vi "12_2.vi"() -> ()   [LabVIEW 2018]
uses:
  <vilib>/Analysis/coordinate.llb/2D Cartesian Coordinate Rotation (Scalar).vi
  <vilib>/Analysis/NI_AALPro.lvlib
panel:
  in  "milliseconds to wait":u32
  out "XY Graph - Light":cluster{"X":dbl, "Y":dbl}[](graph)
  out "Manhattan Distance":dbl
  in  "Input":string="E5\nR90\nE5\nL90\nF80\nL90\nE3\nN5\nF10\nS2\nW1\nF98\nL180\nW1\nF55\nL90\nF73\nN1\nE3\nS2\nE5\nR90\nE2\nS4\nF34\nR90\nW2\nL90\nW4\nF92\nR90\nW4\nN5\nR90\nF73\nS4\nW3\nN4\nR90\nS3\nW3\nN4\nF30\nS5\nE4\nR90\nW5\nR90\nS3\nE5\nL180\nE2\nS4\nE4\nS2\nW3\nF19\nN2\nF53\nR90\nW4\nR90\nN3\nW5\nR90\nW4\nF68\nW4\nN5\nF26\nW4\nF11\nL90\nE5\nL90\nF67\nW3\nS3\nF15\nE4\nS4\nE5\nS1\nF11\nR90\nE3\nF46\nR90\nF40\nE3\nR90\nF35\nR180\nE3\nS5\nL90\nE3\nF63\nE4\nF56\nN2\nE1\nR90\nN3\nF42\nW2\nS4\nN3\nR90\nW2\nR90\nF45\nN5\nL90\nF38\nL90\nN5\nE4\nR90\nN2\nR90\nS4\nR90\nN3\nF53\nR90\nF72\nS5\nE3\nF98\nL90\nE3\nF56\nS2\nF29\nE2\nW3\nL180\nS4\nF31\nS2\nR90\nN5\nR270\nF45\nL90\nF10\nN5\nR90\nE5\nF47\nR90\nS3\nF98\nR90\nF85\nE1\nL90\nS4\nR180\nN4\nL90\nW5\nR90\nE4\nL90\nF24\nR90\nN4\nW3\n..."
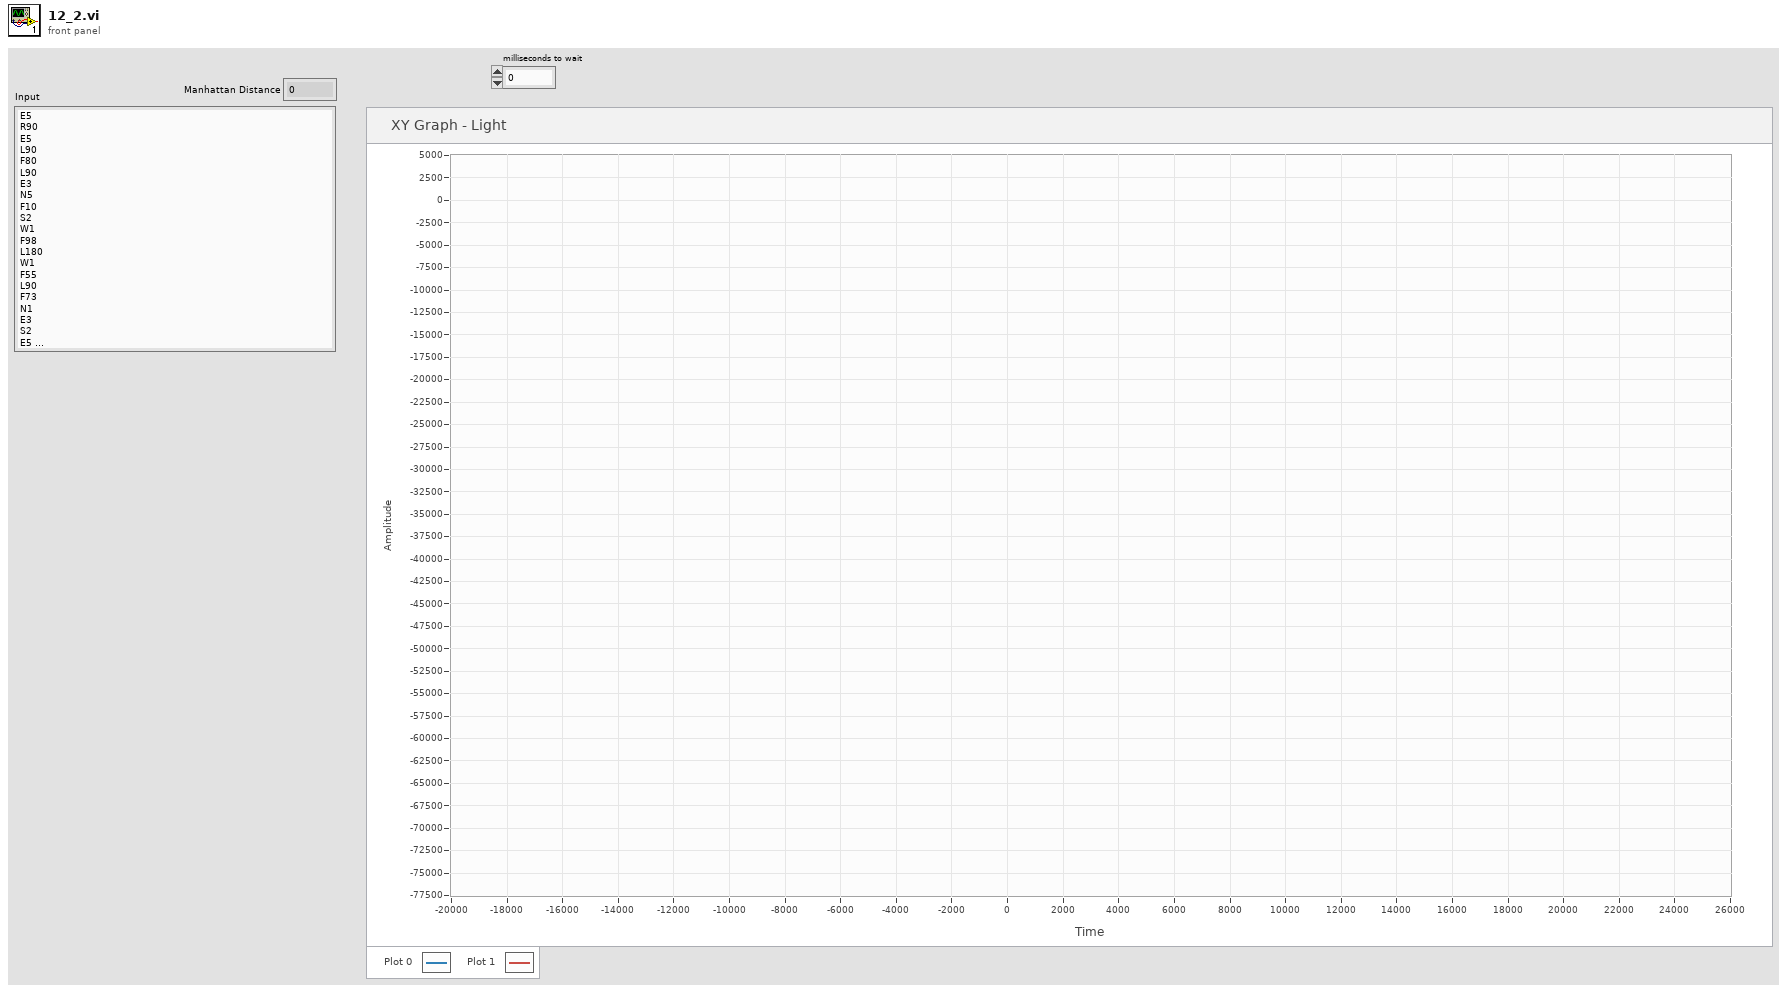
[diagram p1: front panel]
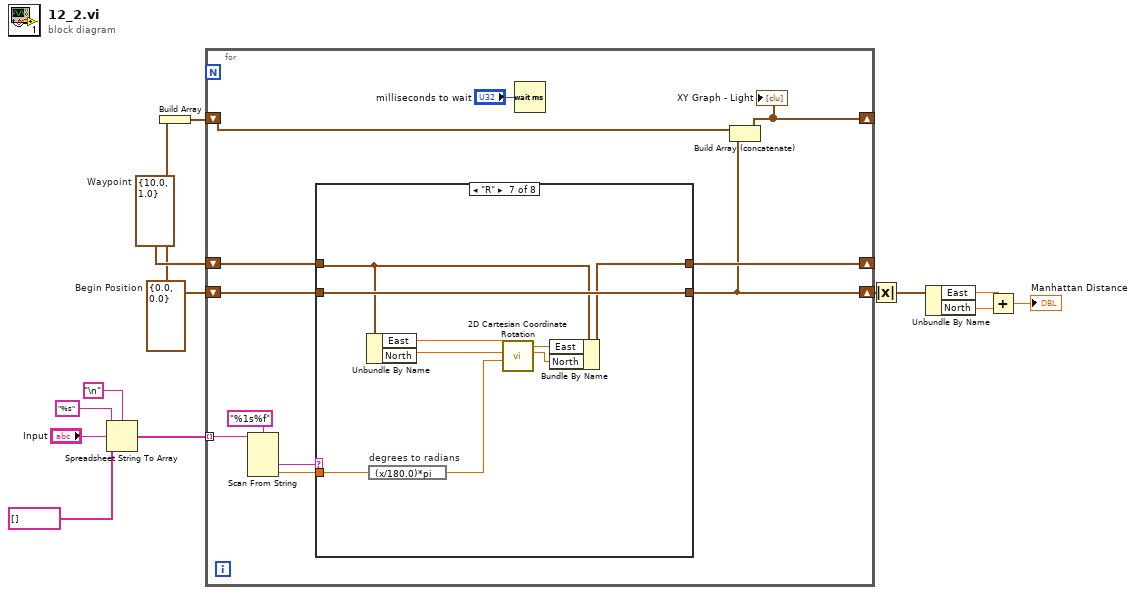
[diagram p0: block diagram]
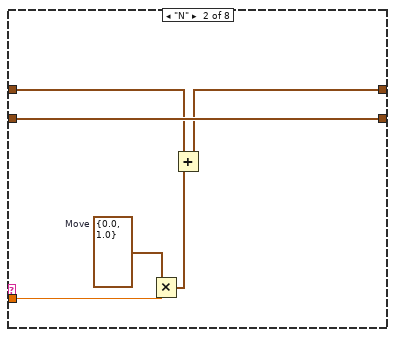
[diagram p3: hidden frame]
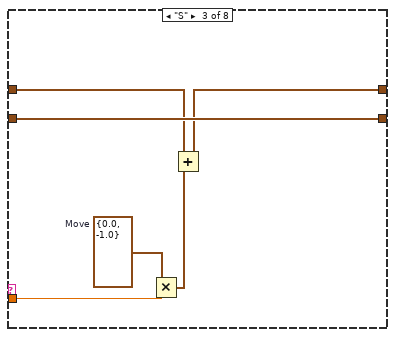
[diagram p4: hidden frame]
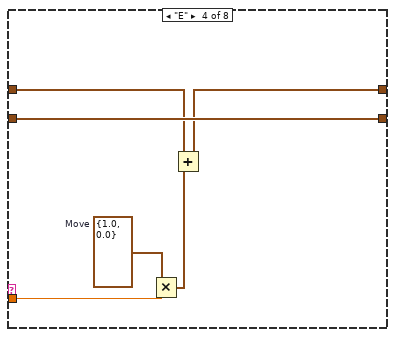
[diagram p5: hidden frame]
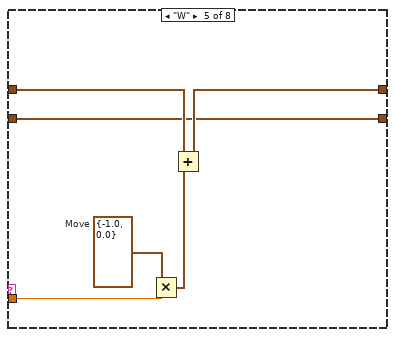
[diagram p6: hidden frame]
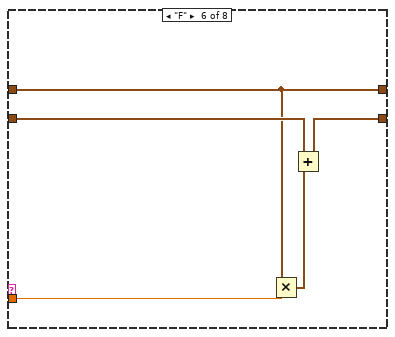
[diagram p7: hidden frame]
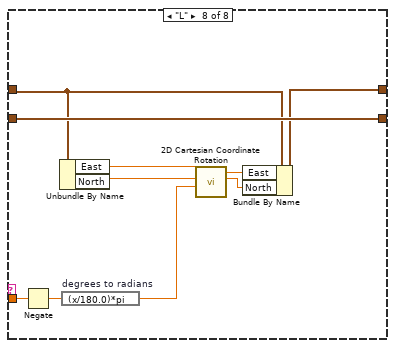
[diagram p8: hidden frame]
diagram:
  w3 = cluster{"East":dbl, "North":dbl} {"East"=10.0, "North"=1.0}  # Waypoint
  w2 = cluster{"East":dbl, "North":dbl} {"East"=0.0, "North"=0.0}  # Begin Position
  n1 = Spreadsheet String To Array(delimiter (Tab)="\n", format string="%s", spreadsheet string="Input", array type (2D Dbl)=string[] []) -> (array=w9:string[])
  n2 = Build Array(w2) -> (w1:cluster{"East":dbl, "North":dbl}[])
  n3 = for {
    tunnel: w9 -> [w24] mode=indexing
    shift-right: [w18] -> _
    shift-left: w3 -> [w21]
    shift-right: [w17] -> w8
    shift-left: w2 -> [w20]
    shift-right: [w16] -> _
    shift-left: w1 -> [w15]
    n4 = Scan From String(format string="%1s%f", input string=w24) -> (output 1=w22:string, output 2=w19:dbl)  [unwired: 4 in, 3 out]
    n5 = case shown="\"R\"" w22 {
      tunnel: w21 -> [w26 w27 w33 w39 w46 w51 w59 w69]
      tunnel: w20 -> [w25 w29 w35 w41 w45 w52 w64 w74]
      tunnel: [w26 w28 w34 w40 w47 w51 w57 w67] -> w18
      tunnel: [w25 w29 w35 w41 w45 w53 w64 w74] -> w17
      tunnel: w19 -> [_ w32 w38 w44 w50 w55 w56 w66]
      frame Default {
      }
      frame "N" {
        w31 = cluster{"East":dbl, "North":dbl} {"East"=0.0, "North"=1.0}  # Move
        n6 = Multiply(x=w31, y=w32) -> (x*y=w30:cluster{"East":dbl, "North":dbl})
        n7 = Add(x=w27, y=w30) -> (x+y=w28:cluster{"East":dbl, "North":dbl})
      }
      frame "S" {
        w37 = cluster{"East":dbl, "North":dbl} {"East"=0.0, "North"=-1.0}  # Move
        n8 = Multiply(x=w37, y=w38) -> (x*y=w36:cluster{"East":dbl, "North":dbl})
        n9 = Add(x=w33, y=w36) -> (x+y=w34:cluster{"East":dbl, "North":dbl})
      }
      frame "E" {
        w43 = cluster{"East":dbl, "North":dbl} {"East"=1.0, "North"=0.0}  # Move
        n10 = Multiply(x=w43, y=w44) -> (x*y=w42:cluster{"East":dbl, "North":dbl})
        n11 = Add(x=w39, y=w42) -> (x+y=w40:cluster{"East":dbl, "North":dbl})
      }
      frame "W" {
        w49 = cluster{"East":dbl, "North":dbl} {"East"=-1.0, "North"=0.0}  # Move
        n12 = Multiply(x=w49, y=w50) -> (x*y=w48:cluster{"East":dbl, "North":dbl})
        n13 = Add(x=w46, y=w48) -> (x+y=w47:cluster{"East":dbl, "North":dbl})
      }
      frame "F" {
        n14 = Multiply(x=w51, y=w55) -> (x*y=w54:cluster{"East":dbl, "North":dbl})
        n15 = Add(x=w52, y=w54) -> (x+y=w53:cluster{"East":dbl, "North":dbl})
      }
      frame "R" {
        n16 = Unbundle By Name(w59) -> ("East"=w62:dbl, "North"=w63:dbl)
        n17 = expression code="(x/180.0)*pi" "degrees to radians"(w56) -> (w61:dbl)
        n18 = call-poly <vilib>:"2D Cartesian Coordinate Rotation.vi"("theta"=w61, "y"=w63, "x"=w62) -> ("y out"=w58:dbl, "x out"=w60:dbl)  [unwired: 6 in, 1 out]
        n19 = Bundle By Name(cluster=w59, "East"=w60, "North"=w58) -> (w57:cluster{"East":dbl, "North":dbl})
      }
      frame "L" {
        n20 = Negate(x=w66) -> (-x=w65:dbl)
        n21 = Unbundle By Name(w69) -> ("East"=w72:dbl, "North"=w73:dbl)
        n22 = expression code="(x/180.0)*pi" "degrees to radians"(w65) -> (w71:dbl)
        n23 = call-poly <vilib>:"2D Cartesian Coordinate Rotation.vi"("theta"=w71, "y"=w73, "x"=w72) -> ("y out"=w68:dbl, "x out"=w70:dbl)  [unwired: 6 in, 1 out]
        n24 = Bundle By Name(cluster=w69, "East"=w70, "North"=w68) -> (w67:cluster{"East":dbl, "North":dbl})
      }
    }
    n25 = Wait (ms)(milliseconds to wait="milliseconds to wait") -> ()  [unwired: 1 out]
    n26 = Build Array (concatenate)(w15, w17) -> (w16:cluster{"East":dbl, "North":dbl}[])
    "XY Graph - Light" <- w16
  }
  n27 = Absolute Value(x=w8) -> (abs(x)=w7:cluster{"East":dbl, "North":dbl})
  n28 = Unbundle By Name(w7) -> ("East"=w5:dbl, "North"=w6:dbl)
  n29 = Add(x=w5, y=w6) -> (x+y=→"Manhattan Distance":dbl)
